vi "Append Properties to Edit Context Menu.vi"(9 "State":T1, 11 "Menu in":refnum<k9>) -> ()   [LabVIEW 2020, in "Stimulus Channel (G3).xctl"]
uses:
  Stimulus Channel (G3).xctl
  State.ctl
  Burst (G3)/Controls.ctl
  Waveform XControls/Waveform (G3)/Waveform (G3).xctl
  Level (G3)/Level (G3).xctl
  Utility VIs/Controls/KRing/KRing.xctl
  Burst (G3)/Burst (G3).xctl
  Level (G3)/Level Units (G3).ctl
  Waveform VIs/Waveform Enum (V3).ctl
  Waveform XControls/Waveform (G3)/Waveform (G3) - Persistent.ctl
  Waveform XControls/Noise (G3)/Noise (G3) - Persistent.ctl
  Calibration VIs/Endpoint VIs/LV Source/Endpoint-Spec.ctl
  Calibration VIs/Endpoint VIs/LV Source/Endpoint-Modality.ctl
  Calibration VIs/Endpoint VIs/LV Source/Endpoint-Laterality.ctl
  Waveform XControls/Noise (G3)/Noise (G3).xctl
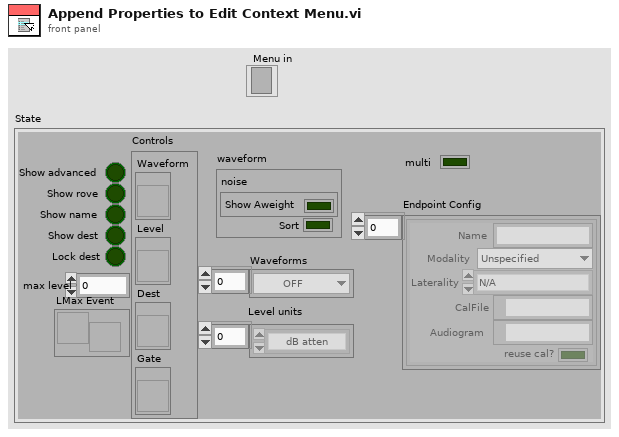
[diagram p1: front panel]
types:
  T1 = typedef "Stimulus Channel (G3).xctl/State.ctl" = cluster{"Show advanced":bool, "Show rove":bool, "Show name":bool, "Show dest":bool, "Lock dest":bool, "max level":dbl, "LMax Event":refnum<user-event>, "Controls":T2, "Level units":T3[], "Waveforms":T4[], "waveform":T5, "Endpoint Config":T7[], "multi":bool}
  T2 = typedef "Controls.ctl" = cluster{"Waveform":refnum<vi>, "Level":refnum<vi>, "Dest":refnum<vi>, "Gate":refnum<vi>}
  T3 = typedef "Level (G3).xctl/Level Units (G3).ctl" = enum16{"dB atten", "dB SPL", "dB re 1 Vrms", "dB V/Hz½", "mW", "dB HL", "Volts", "dB mW"}
  T4 = typedef "Waveform Enum (V3).ctl" = enum16{"OFF", "Tone", "Noise", "Pulse Train", "File", "FM Sweep", "Chirp Train", "Complex Tone", "FM Tone", "Vowel", "Ramp"}
  T5 = typedef "Waveform (G3).xctl/Waveform (G3) - Persistent.ctl" = cluster{"noise":T6, "Sort":bool}
  T6 = typedef "Noise (G3).xctl/Noise (G3) - Persistent.ctl" = cluster{"Show Aweight":bool}
  T7 = typedef "Endpoint-Spec.ctl" = cluster{"Name":string, "Modality":T8, "Laterality":T9, "CalFile":path, "Audiogram":path, "reuse cal?":bool}
  T8 = typedef "Endpoint-Modality.ctl" = enum16{"Unspecified", "Acoustic", "Electric", "Optical"}
  T9 = typedef "Endpoint-Laterality.ctl" = enum16{"N/A", "Right", "Left"}
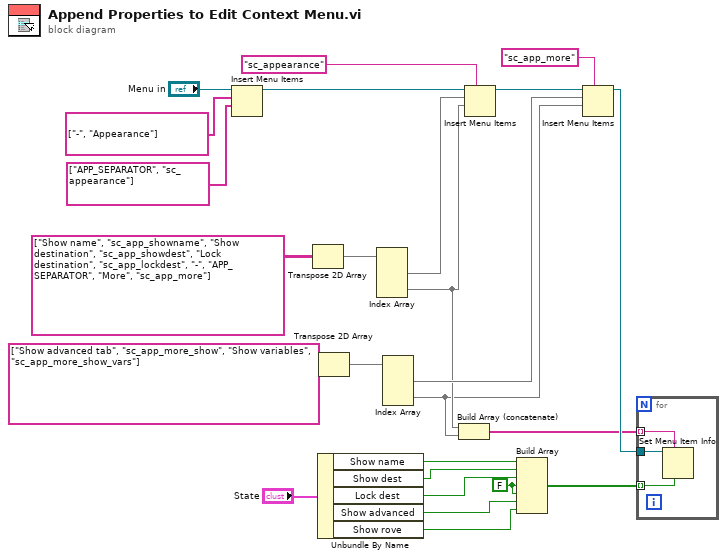
[diagram p0: block diagram]
diagram:
  w1 = FALSE ("element")
  n1 = Insert Menu Items(7:string[] ["APP_SEPARATOR", "sc_appearance"] ("item names"), 8:string[] ["-", "Appearance"] ("item names"), 9:"Menu in") -> (3:w24:refnum<k9>)  [unwired: 3 in, 2 out]
  n2 = Transpose 2D Array(2D array=string[][] [["Show name", "sc_app_showname"], ["Show destination", "sc_app_showdest"], ["Lock destination", "sc_app_lockdest"], ["-", "APP_SEPARATOR"], ["More", "sc_app_more"]] ("item names")) -> (transposed array=w19:string[][])
  n3 = Unbundle By Name("State") -> ("Show name"=w9:bool, "Show dest"=w8:bool, "Lock dest"=w7:bool, "Show advanced"=w6:bool, "Show rove"=w5:bool)
  n4 = Transpose 2D Array(2D array=string[][] [["Show advanced tab", "sc_app_more_show"], ["Show variables", "sc_app_more_show_vars"]] ("item names")) -> (transposed array=w14:string[][])
  n5 = Index Array(array=w19) -> (element #1=w18:string[], element #2=w11:string[])  [unwired: 4 in]
  n6 = Index Array(array=w14) -> (element #1=w13:string[], element #2=w10:string[])  [unwired: 4 in]
  n7 = Build Array (concatenate)(w11, w10) -> (w2:string[])
  n8 = Insert Menu Items(5:"sc_appearance", 7:w11, 8:w18, 9:w24) -> (3:w16:refnum<k9>)  [unwired: 2 in, 2 out]
  n9 = Build Array(w9, w8, w7, w1, w1, w6, w5) -> (w3:bool[])
  n10 = Insert Menu Items(5:"sc_app_more", 7:w10, 8:w13, 9:w16) -> (3:w4:refnum<k9>)  [unwired: 2 in, 2 out]
  n11 = for {
    tunnel: w4 -> [w28]
    tunnel: w3 -> [w27] mode=indexing
    tunnel: w2 -> [w26] mode=indexing
    n12 = Set Menu Item Info(6:w27, 7:w26, 11:w28) -> ()  [unwired: 4 in, 2 out]
  }
